vi "input.vi"(8 "error in":errorcluster, 10 "data table in":T1, 11 "OPC UA runtime in":refnum<class "OPC UA runtime.lvclass">) -> (0 "error out":errorcluster, 2 "data table out":T1, 3 "OPC UA runtime out":refnum<class "OPC UA runtime.lvclass">)   [LabVIEW 2013, in "OPC UA runtime.lvclass"]
doc: "Provides an interface for reading data from a module at runtime. While this interface performs no operations, a child should provide an override which may read from any open sessions, references, or interfaces."
uses:
  OPC UA runtime.lvclass
  <vilib>/NI/Tag Bus/table/data table.lvlib
  <vilib>/opcua/NI OPC UA Client.lvlib
  <vilib>/OPCUA/client/Read Bool.vi
  <vilib>/NI/Tag Bus/table/data polymorphs/write one/write Boolean.vi
  <vilib>/NI/Tag Bus/table/data polymorphs/write one/write String.vi
  <vilib>/NI/Tag Bus/table/data polymorphs/write one/write Array of String.vi
  <vilib>/OPCUA/client/Read UInt16.vi
  <vilib>/OPCUA/client/Read Int32.vi
  <vilib>/OPCUA/client/Read ByteString Array.vi
  <vilib>/OPCUA/client/Read SByte.vi
  <vilib>/OPCUA/client/Read String Array.vi
  <vilib>/OPCUA/client/Read UInt32.vi
  <vilib>/OPCUA/client/Read Double.vi
  <vilib>/OPCUA/client/Read Float.vi
  <vilib>/OPCUA/client/Read Int64.vi
  <vilib>/OPCUA/client/Read UInt64.vi
  <vilib>/OPCUA/client/Read Double Array.vi
  <vilib>/OPCUA/client/Read Int16 Array.vi
  <vilib>/OPCUA/client/Read Byte Array.vi
  <vilib>/OPCUA/client/Read UInt64 Array.vi
  <vilib>/OPCUA/client/Read Int32 Array.vi
  <vilib>/OPCUA/client/Read ByteString.vi
  <vilib>/OPCUA/client/Read UInt32 Array.vi
  <vilib>/OPCUA/client/Read SByte Array.vi
  <vilib>/OPCUA/client/Read UInt16 Array.vi
  <vilib>/OPCUA/client/Read Int16.vi
  <vilib>/OPCUA/client/Read String.vi
  <vilib>/OPCUA/client/Read Int64 Array.vi
  <vilib>/OPCUA/client/Read Byte.vi
  <vilib>/OPCUA/client/Read Float Array.vi
  <vilib>/OPCUA/client/Read Bool Array.vi
  <vilib>/NI/Tag Bus/table/data polymorphs/write one/write I16.vi
  <vilib>/NI/Tag Bus/table/data polymorphs/write one/write U16.vi
  <vilib>/NI/Tag Bus/table/data polymorphs/write one/write I32.vi
  <vilib>/NI/Tag Bus/table/data polymorphs/write one/write Array of I64.vi
  <vilib>/NI/Tag Bus/table/data polymorphs/write one/write Array of I16.vi
  <vilib>/NI/Tag Bus/table/data polymorphs/write one/write Single.vi
  <vilib>/NI/Tag Bus/table/data polymorphs/write one/write I64.vi
  <vilib>/NI/Tag Bus/table/data polymorphs/write one/write U32.vi
  <vilib>/NI/Tag Bus/table/data polymorphs/write one/write U64.vi
  <vilib>/NI/Tag Bus/table/data polymorphs/write one/write U8.vi
  <vilib>/NI/Tag Bus/table/data polymorphs/write one/write Array of I8.vi
  <vilib>/NI/Tag Bus/table/data polymorphs/write one/write Array of U16.vi
  <vilib>/NI/Tag Bus/table/data polymorphs/write one/write I8.vi
  <vilib>/NI/Tag Bus/table/data polymorphs/write one/write Array of U32.vi
  <vilib>/NI/Tag Bus/table/data polymorphs/write one/write Array of I32.vi
  <vilib>/NI/Tag Bus/table/data polymorphs/write one/write Array of Boolean.vi
  <vilib>/NI/Tag Bus/table/data polymorphs/write one/write Array of U8.vi
  <vilib>/NI/Tag Bus/table/data polymorphs/write one/write Array of Single.vi
  <vilib>/NI/Tag Bus/table/data polymorphs/write one/write Array of Double.vi
  <vilib>/NI/Tag Bus/table/data polymorphs/write one/write Array of U64.vi
  <vilib>/NI/Tag Bus/table/data polymorphs/write one/write Double.vi
  <vilib>/OPCUA/client/Read DateTime.vi
  <vilib>/OPCUA/client/Read DateTime Array.vi
  <vilib>/opcua/NI OPC UA Server.lvlib
  <vilib>/OPCUA/server/Read Bool.vi
  <vilib>/OPCUA/server/Read SByte.vi
  <vilib>/OPCUA/server/Read Byte.vi
  <vilib>/OPCUA/server/Read Int16.vi
  <vilib>/OPCUA/server/Read UInt16.vi
  <vilib>/OPCUA/server/Read Int32.vi
  <vilib>/OPCUA/server/Read UInt32.vi
  <vilib>/OPCUA/server/Read Int64.vi
  <vilib>/OPCUA/server/Read UInt64.vi
  <vilib>/OPCUA/server/Read Float.vi
  <vilib>/OPCUA/server/Read Double.vi
  <vilib>/OPCUA/server/Read String.vi
  <vilib>/OPCUA/server/Read Date Time.vi
  <vilib>/OPCUA/server/Read Byte String.vi
  <vilib>/OPCUA/server/Read Bool Array.vi
  <vilib>/OPCUA/server/Read SByte Array.vi
  <vilib>/OPCUA/server/Read Byte Array.vi
  <vilib>/OPCUA/server/Read Int16 Array.vi
  <vilib>/OPCUA/server/Read UInt16 Array.vi
  <vilib>/OPCUA/server/Read Int32 Array.vi
  <vilib>/OPCUA/server/Read UInt32 Array.vi
  <vilib>/OPCUA/server/Read Int64 Array.vi
  <vilib>/OPCUA/server/Read UInt64 Array.vi
  <vilib>/OPCUA/server/Read Float Array.vi
  <vilib>/OPCUA/server/Read Double Array.vi
  <vilib>/OPCUA/server/Read String Array.vi
  <vilib>/OPCUA/server/Read Date Time Array.vi
  <vilib>/OPCUA/server/Read Byte String Array.vi
  <vilib>/NI/Tag Bus/table/data table.ctl
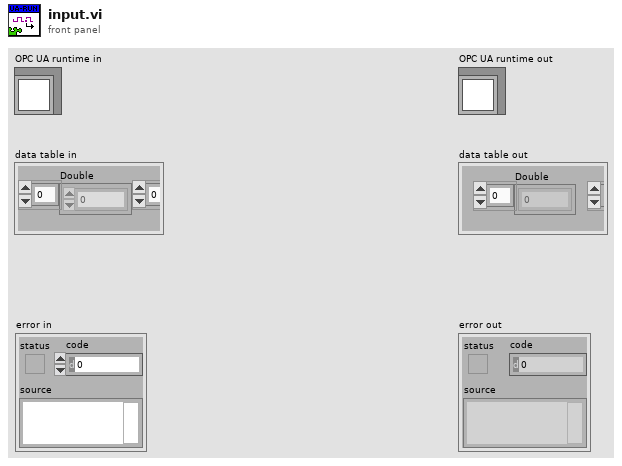
[diagram p1: front panel]
types:
  T1 = typedef "tag bus.lvlib/data table.lvlib/data table.ctl" = cluster{"Double":dbl[], "Single":sgl[], "I64":i64[], "I32":i32[], "I16":i16[], "I8":i8[], "U64":u64[], "U32":u32[], "U16":u16[], "U8":u8[], "Boolean":bool[], "String":string[], "Array of Double":cluster{"DBL Array":dbl[]}[], "Array of Single":cluster{"SGL Array":sgl[]}[], "Array of I64":cluster{"I64 Array":i64[]}[], "Array of I32":cluster{"I32 Array":i32[]}[], "Array of I16":cluster{"I16 Array":i16[]}[], "Array of I8":cluster{"I8 Array":i8[]}[], "Array of U64":cluster{"U64 Array":u64[]}[], "Array of U32":cluster{"U32 Array":u32[]}[], "Array of U16":cluster{"U16 Array":u16[]}[], "Array of U8":cluster{"U8 Array":u8[]}[], "Array of Boolean":cluster{"Boolean Array":bool[]}[], "Array of String":cluster{"String Array":string[]}[]}
  T2 = typedef "tag bus.lvlib/tag descriptor.lvclass/Data Type.ctl" = enum16{"Double", "Single", "I64", "I32", "I16", "I8", "U64", "U32", "U16", "U8", "Boolean", "String", "Array of Double", "Array of Single", "Array of I64", "Array of I32", "Array of I16", "Array of I8", "Array of U64", "Array of U32", "Array of U16", "Array of U8", "Array of Boolean", "Array of String"}
  T3 = typedef "OPC UA configuration.lvclass/OPC UA Data Type.ctl" = u16
  T4 = cluster{"DCAF Data Type":T2, "Index":i32, "Node Path":string, "OPC UA Data Type":T3}[]
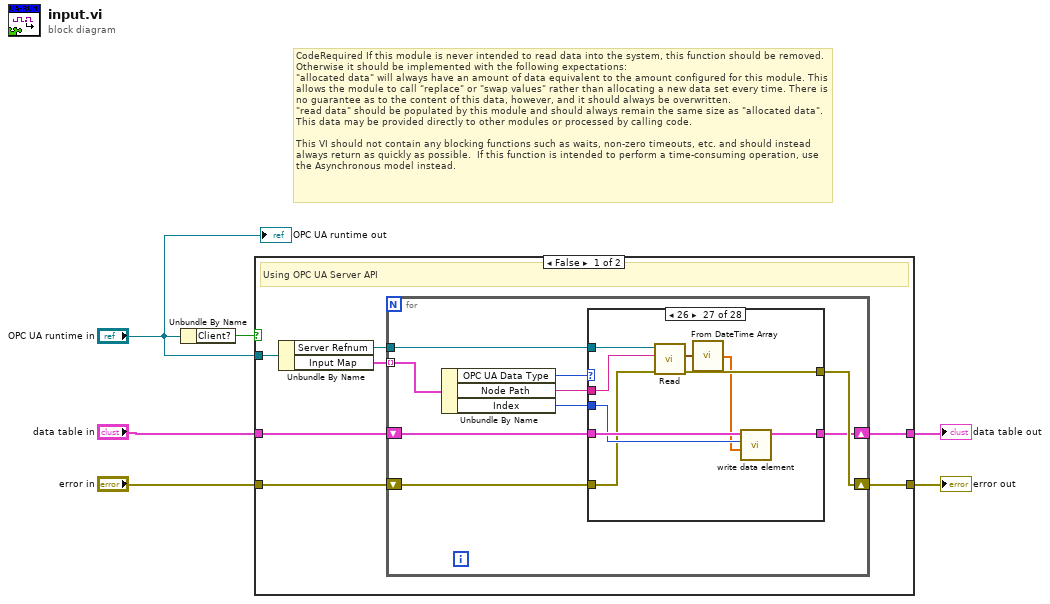
[diagram p0: block diagram]
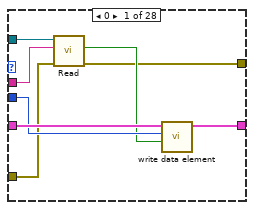
[diagram p2: hidden frame]
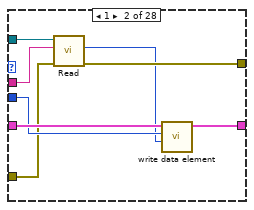
[diagram p3: hidden frame]
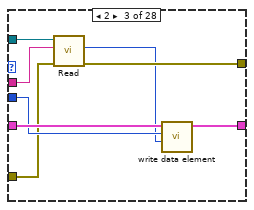
[diagram p4: hidden frame]
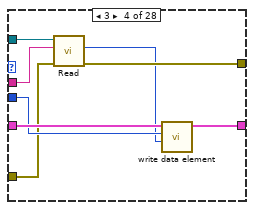
[diagram p5: hidden frame]
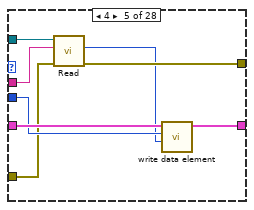
[diagram p6: hidden frame]
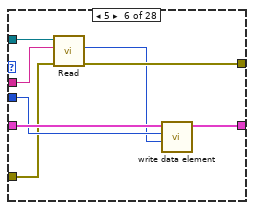
[diagram p7: hidden frame]
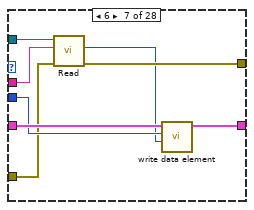
[diagram p8: hidden frame]
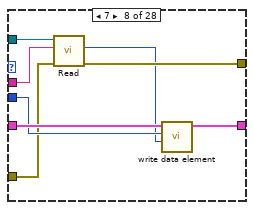
[diagram p9: hidden frame]
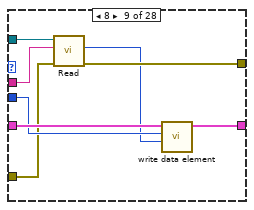
[diagram p10: hidden frame]
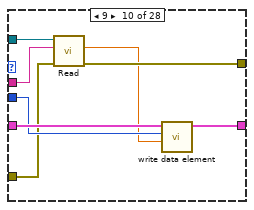
[diagram p11: hidden frame]
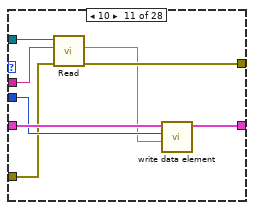
[diagram p12: hidden frame]
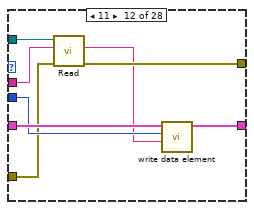
[diagram p13: hidden frame]
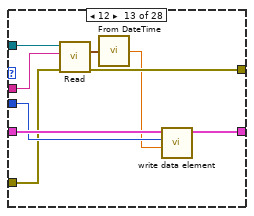
[diagram p14: hidden frame]
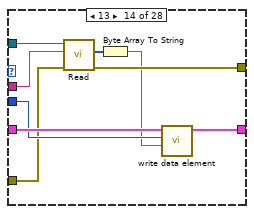
[diagram p15: hidden frame]
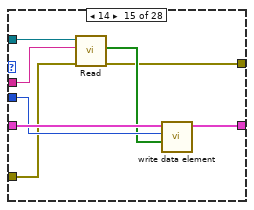
[diagram p16: hidden frame]
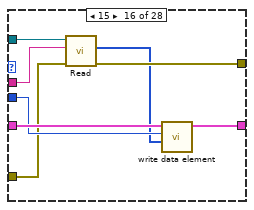
[diagram p17: hidden frame]
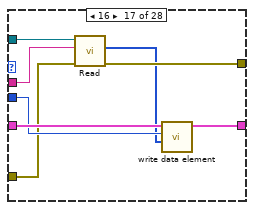
[diagram p18: hidden frame]
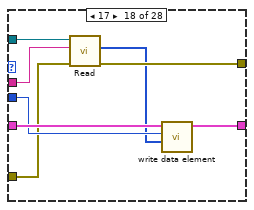
[diagram p19: hidden frame]
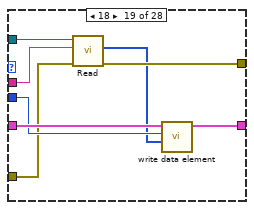
[diagram p20: hidden frame]
diagram:
  # "CodeRequired If this module is never intended to read data into the system, this function should be removed. Otherwise it should be implemented with the following expectations:\n\"allocated data\" will always have an amount of data equivalent to the amount configured for this module. This allows the module to call \"replace\" or \"swap values\" rather than allocating a new data set every time. There is no guarantee as to the content of this data, however, and it should always be overwritten.\n\"read data\" should be populated by this module and should always remain the same size as \"allocated data\". This data may be provided directly to other modules or processed by calling code.\n\nThis VI should not contain any blocking functions such as waits, non-zero timeouts, etc. and should instead always return as quickly as possible.  If this function is intended to perform a time-consuming operation, use the Asynchronous model instead."
  n1 = Unbundle By Name("OPC UA runtime in") -> ("Client?"=w6:bool)
  n2 = case shown="False" w6 {
    tunnel: "OPC UA runtime in" -> [w13 w259]
    tunnel: "data table in" -> [w9 w256]
    tunnel: "error in" -> [w8 w255]
    tunnel: [w10 w254] -> w2
    tunnel: [w7 w253] -> w1
    frame False {
      # "Using OPC UA Server API"
      n3 = Unbundle By Name(w13) -> ("Server Refnum"=w11:refnum<k21>, "Input Map"=w12:T4)
      n4 = for {
        tunnel: w11 -> [w18]
        tunnel: w12 -> [w22] mode=indexing
        shift-right: [w15] -> w7
        shift-left: w8 -> [w16]
        shift-right: [w14] -> w10
        shift-left: w9 -> [w17]
        n5 = Unbundle By Name(w22) -> ("OPC UA Data Type"=w21:T3, "Node Path"=w20:string, "Index"=w19:i32)
        n6 = case shown="26" w21 {
          tunnel: w20 -> [w29 w37 w45 w53 w61 w69 w77 w85 w93 w101 w109 w117 w126 w135 w144 w152 w160 w168 w176 w184 w192 w200 w208 w216 w224 w232 w241 w249]
          tunnel: w19 -> [w27 w35 w43 w51 w59 w67 w75 w83 w91 w99 w107 w115 w124 w133 w142 w150 w158 w166 w174 w182 w190 w198 w206 w214 w222 w230 w239 w247]
          tunnel: w18 -> [w30 w38 w46 w54 w62 w70 w78 w86 w94 w102 w110 w118 w127 w136 w137 w146 w153 w162 w170 w178 w186 w194 w202 w210 w218 w225 w234 w250]
          tunnel: w17 -> [w28 w36 w44 w52 w60 w68 w76 w84 w92 w100 w108 w116 w125 w134 w143 w151 w159 w167 w175 w183 w191 w199 w207 w215 w223 w231 w240 w248]
          tunnel: w16 -> [w25 w34 w42 w50 w58 w66 w74 w82 w90 w98 w106 w114 w123 w132 w140 w149 w157 w165 w173 w181 w189 w197 w205 w213 w221 w228 w238 w246]
          tunnel: [w24 w33 w41 w49 w57 w65 w73 w81 w89 w97 w105 w113 w122 w131 w139 w148 w156 w164 w172 w180 w188 w196 w204 w212 w220 w227 w237 w245] -> w15
          tunnel: [w23 w32 w40 w48 w56 w64 w72 w80 w88 w96 w104 w112 w121 w130 w138 w147 w155 w163 w171 w179 w187 w195 w203 w211 w219 w226 w236 w244] -> w14
          frame 0 {
            n7 = call-poly <vilib>:"Read.vi"("error in (no error)"=w25, "node path"=w29, "OPC UA server refnum in"=w30) -> ("error out"=w24:errorcluster, "value"=w26:bool)  [unwired: 4 in, 3 out]
            n8 = call-poly <vilib>:"write data element.vi"("value"=w26, "index"=w27, "data table in"=w28) -> ("data table out"=w23:T1)  [unwired: 8 in]
          }
          frame 1 {
            n9 = call-poly <vilib>:"Read.vi"("error in (no error)"=w34, "node path"=w37, "OPC UA server refnum in"=w38) -> ("error out"=w33:errorcluster, "value"=w31:i8)  [unwired: 4 in, 3 out]
            n10 = call-poly <vilib>:"write data element.vi"("value"=w31, "index"=w35, "data table in"=w36) -> ("data table out"=w32:T1)  [unwired: 8 in]
          }
          frame 2 {
            n11 = call-poly <vilib>:"Read.vi"("error in (no error)"=w42, "node path"=w45, "OPC UA server refnum in"=w46) -> ("error out"=w41:errorcluster, "value"=w39:u8)  [unwired: 4 in, 3 out]
            n12 = call-poly <vilib>:"write data element.vi"("value"=w39, "index"=w43, "data table in"=w44) -> ("data table out"=w40:T1)  [unwired: 8 in]
          }
          frame 3 {
            n13 = call-poly <vilib>:"Read.vi"("error in (no error)"=w50, "node path"=w53, "OPC UA server refnum in"=w54) -> ("error out"=w49:errorcluster, "value"=w47:i16)  [unwired: 4 in, 3 out]
            n14 = call-poly <vilib>:"write data element.vi"("value"=w47, "index"=w51, "data table in"=w52) -> ("data table out"=w48:T1)  [unwired: 8 in]
          }
          frame 4 {
            n15 = call-poly <vilib>:"Read.vi"("error in (no error)"=w58, "node path"=w61, "OPC UA server refnum in"=w62) -> ("error out"=w57:errorcluster, "value"=w55:u16)  [unwired: 4 in, 3 out]
            n16 = call-poly <vilib>:"write data element.vi"("value"=w55, "index"=w59, "data table in"=w60) -> ("data table out"=w56:T1)  [unwired: 8 in]
          }
          frame 5 {
            n17 = call-poly <vilib>:"Read.vi"("error in (no error)"=w66, "node path"=w69, "OPC UA server refnum in"=w70) -> ("error out"=w65:errorcluster, "value"=w63:i32)  [unwired: 4 in, 3 out]
            n18 = call-poly <vilib>:"write data element.vi"("value"=w63, "index"=w67, "data table in"=w68) -> ("data table out"=w64:T1)  [unwired: 8 in]
          }
          frame 6 {
            n19 = call-poly <vilib>:"Read.vi"("error in (no error)"=w74, "node path"=w77, "OPC UA server refnum in"=w78) -> ("error out"=w73:errorcluster, "value"=w71:u32)  [unwired: 4 in, 3 out]
            n20 = call-poly <vilib>:"write data element.vi"("value"=w71, "index"=w75, "data table in"=w76) -> ("data table out"=w72:T1)  [unwired: 8 in]
          }
          frame 7 {
            n21 = call-poly <vilib>:"Read.vi"("error in (no error)"=w82, "node path"=w85, "OPC UA server refnum in"=w86) -> ("error out"=w81:errorcluster, "value"=w79:i64)  [unwired: 4 in, 3 out]
            n22 = call-poly <vilib>:"write data element.vi"("value"=w79, "index"=w83, "data table in"=w84) -> ("data table out"=w80:T1)  [unwired: 8 in]
          }
          frame 8 {
            n23 = call-poly <vilib>:"Read.vi"("error in (no error)"=w90, "node path"=w93, "OPC UA server refnum in"=w94) -> ("error out"=w89:errorcluster, "value"=w87:u64)  [unwired: 4 in, 3 out]
            n24 = call-poly <vilib>:"write data element.vi"("value"=w87, "index"=w91, "data table in"=w92) -> ("data table out"=w88:T1)  [unwired: 8 in]
          }
          frame 9 {
            n25 = call-poly <vilib>:"Read.vi"("error in (no error)"=w98, "node path"=w101, "OPC UA server refnum in"=w102) -> ("error out"=w97:errorcluster, "value"=w95:sgl)  [unwired: 4 in, 3 out]
            n26 = call-poly <vilib>:"write data element.vi"("value"=w95, "index"=w99, "data table in"=w100) -> ("data table out"=w96:T1)  [unwired: 8 in]
          }
          frame 10 {
            n27 = call-poly <vilib>:"Read.vi"("error in (no error)"=w106, "node path"=w109, "OPC UA server refnum in"=w110) -> ("error out"=w105:errorcluster, "value"=w103:dbl)  [unwired: 4 in, 3 out]
            n28 = call-poly <vilib>:"write data element.vi"("value"=w103, "index"=w107, "data table in"=w108) -> ("data table out"=w104:T1)  [unwired: 8 in]
          }
          frame 11 {
            n29 = call-poly <vilib>:"Read.vi"("error in (no error)"=w114, "node path"=w117, "OPC UA server refnum in"=w118) -> ("error out"=w113:errorcluster, "value"=w111:string)  [unwired: 4 in, 3 out]
            n30 = call-poly <vilib>:"write data element.vi"("value"=w111, "index"=w115, "data table in"=w116) -> ("data table out"=w112:T1)  [unwired: 8 in]
          }
          frame 12 {
            n31 = call-poly <vilib>:"Read.vi"("error in (error in)"=w123, "node path"=w126, "OPC UA server refnum in"=w127) -> ("error out"=w122:errorcluster, "timestamp"=w120:timestamp)  [unwired: 4 in, 3 out]
            n32 = call "From DateTime.vi"("DateTime"=w120) -> ("Formatted DateTime"=w119:dbl)
            n33 = call-poly <vilib>:"write data element.vi"("value"=w119, "index"=w124, "data table in"=w125) -> ("data table out"=w121:T1)  [unwired: 8 in]
          }
          frame 13 {
            n34 = call-poly <vilib>:"Read.vi"("error in (no error)"=w132, "node path"=w135, "OPC UA server refnum in"=w136) -> ("error out"=w131:errorcluster, "value"=w128:u8[])  [unwired: 4 in, 3 out]
            n35 = Byte Array To String(unsigned byte array=w128) -> (string=w129:string)
            n36 = call-poly <vilib>:"write data element.vi"("value"=w129, "index"=w133, "data table in"=w134) -> ("data table out"=w130:T1)  [unwired: 8 in]
          }
          frame 14 {
            n37 = call-poly <vilib>:"Read.vi"("error in (no error)"=w140, "node path"=w144, "OPC UA server refnum in"=w137) -> ("error out"=w139:errorcluster, "value"=w141:bool[])  [unwired: 4 in, 3 out]
            n38 = call-poly <vilib>:"write data element.vi"("value"=w141, "index"=w142, "data table in"=w143) -> ("data table out"=w138:T1)  [unwired: 8 in]
          }
          frame 15 {
            n39 = call-poly <vilib>:"Read.vi"("error in (no error)"=w149, "node path"=w152, "OPC UA server refnum in"=w146) -> ("error out"=w148:errorcluster, "value"=w145:i8[])  [unwired: 4 in, 3 out]
            n40 = call-poly <vilib>:"write data element.vi"("value"=w145, "index"=w150, "data table in"=w151) -> ("data table out"=w147:T1)  [unwired: 8 in]
          }
          frame 16 {
            n41 = call-poly <vilib>:"Read.vi"("error in (no error)"=w157, "node path"=w160, "OPC UA server refnum in"=w153) -> ("error out"=w156:errorcluster, "value"=w154:u8[])  [unwired: 4 in, 3 out]
            n42 = call-poly <vilib>:"write data element.vi"("value"=w154, "index"=w158, "data table in"=w159) -> ("data table out"=w155:T1)  [unwired: 8 in]
          }
          frame 17 {
            n43 = call-poly <vilib>:"Read.vi"("error in (no error)"=w165, "node path"=w168, "OPC UA server refnum in"=w162) -> ("error out"=w164:errorcluster, "value"=w161:i16[])  [unwired: 4 in, 3 out]
            n44 = call-poly <vilib>:"write data element.vi"("value"=w161, "index"=w166, "data table in"=w167) -> ("data table out"=w163:T1)  [unwired: 8 in]
          }
          frame 18 {
            n45 = call-poly <vilib>:"Read.vi"("error in (no error)"=w173, "node path"=w176, "OPC UA server refnum in"=w170) -> ("error out"=w172:errorcluster, "value"=w169:u16[])  [unwired: 4 in, 3 out]
            n46 = call-poly <vilib>:"write data element.vi"("value"=w169, "index"=w174, "data table in"=w175) -> ("data table out"=w171:T1)  [unwired: 8 in]
          }
          frame 19 {
            n47 = call-poly <vilib>:"Read.vi"("error in (no error)"=w181, "node path"=w184, "OPC UA server refnum in"=w178) -> ("error out"=w180:errorcluster, "value"=w177:i32[])  [unwired: 4 in, 3 out]
            n48 = call-poly <vilib>:"write data element.vi"("value"=w177, "index"=w182, "data table in"=w183) -> ("data table out"=w179:T1)  [unwired: 8 in]
          }
          frame 20 {
            n49 = call-poly <vilib>:"Read.vi"("error in (no error)"=w189, "node path"=w192, "OPC UA server refnum in"=w186) -> ("error out"=w188:errorcluster, "value"=w185:u32[])  [unwired: 4 in, 3 out]
            n50 = call-poly <vilib>:"write data element.vi"("value"=w185, "index"=w190, "data table in"=w191) -> ("data table out"=w187:T1)  [unwired: 8 in]
          }
          frame 21 {
            n51 = call-poly <vilib>:"Read.vi"("error in (no error)"=w197, "node path"=w200, "OPC UA server refnum in"=w194) -> ("error out"=w196:errorcluster, "value"=w193:i64[])  [unwired: 4 in, 3 out]
            n52 = call-poly <vilib>:"write data element.vi"("value"=w193, "index"=w198, "data table in"=w199) -> ("data table out"=w195:T1)  [unwired: 8 in]
          }
          frame 22 {
            n53 = call-poly <vilib>:"Read.vi"("error in (no error)"=w205, "node path"=w208, "OPC UA server refnum in"=w202) -> ("error out"=w204:errorcluster, "value"=w201:u64[])  [unwired: 4 in, 3 out]
            n54 = call-poly <vilib>:"write data element.vi"("value"=w201, "index"=w206, "data table in"=w207) -> ("data table out"=w203:T1)  [unwired: 8 in]
          }
          frame 23 {
            n55 = call-poly <vilib>:"Read.vi"("error in (no error)"=w213, "node path"=w216, "OPC UA server refnum in"=w210) -> ("error out"=w212:errorcluster, "value"=w209:sgl[])  [unwired: 4 in, 3 out]
            n56 = call-poly <vilib>:"write data element.vi"("value"=w209, "index"=w214, "data table in"=w215) -> ("data table out"=w211:T1)  [unwired: 8 in]
          }
          frame 24 {
            n57 = call-poly <vilib>:"Read.vi"("error in (no error)"=w221, "node path"=w224, "OPC UA server refnum in"=w218) -> ("error out"=w220:errorcluster, "value"=w217:dbl[])  [unwired: 4 in, 3 out]
            n58 = call-poly <vilib>:"write data element.vi"("value"=w217, "index"=w222, "data table in"=w223) -> ("data table out"=w219:T1)  [unwired: 8 in]
          }
          frame 25 {
            n59 = call-poly <vilib>:"Read.vi"("error in (no error)"=w228, "node path"=w232, "OPC UA server refnum in"=w225) -> ("error out"=w227:errorcluster, "value"=w229:string[])  [unwired: 4 in, 3 out]
            n60 = call-poly <vilib>:"write data element.vi"("value"=w229, "index"=w230, "data table in"=w231) -> ("data table out"=w226:T1)  [unwired: 8 in]
          }
          frame 26 {
            n61 = call-poly <vilib>:"Read.vi"("error in (no error)"=w238, "node path"=w241, "OPC UA server refnum in"=w234) -> ("error out"=w237:errorcluster, "value"=w233:timestamp[])  [unwired: 4 in, 3 out]
            n62 = call "From DateTime Array.vi"("DateTime Array"=w233) -> ("Formatted DateTime Array"=w235:dbl[])
            n63 = call-poly <vilib>:"write data element.vi"("value"=w235, "index"=w239, "data table in"=w240) -> ("data table out"=w236:T1)  [unwired: 8 in]
          }
          frame 27 {
            n64 = call-poly <vilib>:"Read.vi"("error in (no error)"=w246, "node path"=w249, "OPC UA server refnum in"=w250) -> ("error out"=w245:errorcluster, "value"=w242:u8[][])  [unwired: 4 in, 3 out]
            n65 = for {
              tunnel: [w252] -> w243 mode=indexing
              tunnel: w242 -> [w251] mode=indexing
              n66 = Byte Array To String(unsigned byte array=w251) -> (string=w252:string)
            }
            n67 = call-poly <vilib>:"write data element.vi"("value"=w243, "index"=w247, "data table in"=w248) -> ("data table out"=w244:T1)  [unwired: 8 in]
          }
        }
      }
    }
    frame True {
      # "Using OPC UA Client API"
      n68 = Unbundle By Name(w259) -> ("Client Refnum"=w258:refnum<k21>, "Input Map"=w257:T4)
      n69 = for {
        tunnel: w258 -> [w264]
        tunnel: w257 -> [w268] mode=indexing
        shift-right: [w261] -> w253
        shift-left: w255 -> [w262]
        shift-right: [w260] -> w254
        shift-left: w256 -> [w263]
        n70 = Unbundle By Name(w268) -> ("OPC UA Data Type"=w267:T3, "Node Path"=w266:string, "Index"=w265:i32)
        n71 = case shown="1" w267 {
          tunnel: w266 -> [w275 w283 w291 w299 w307 w315 w323 w331 w339 w347 w355 w363 w372 w381 w389 w397 w405 w413 w421 w429 w437 w445 w453 w461 w469 w477 w486 w495]
          tunnel: w265 -> [w273 w281 w289 w297 w305 w313 w321 w329 w337 w345 w353 w361 w370 w379 w387 w395 w403 w411 w419 w427 w435 w443 w451 w459 w467 w475 w484 w493]
          tunnel: w264 -> [w276 w284 w292 w300 w308 w316 w324 w332 w340 w348 w356 w364 w373 w382 w390 w398 w406 w414 w422 w430 w438 w446 w454 w462 w470 w478 w487 w496]
          tunnel: w263 -> [w274 w282 w290 w298 w306 w314 w322 w330 w338 w346 w354 w362 w371 w380 w388 w396 w404 w412 w420 w428 w436 w444 w452 w460 w468 w476 w485 w494]
          tunnel: w262 -> [w271 w279 w287 w295 w303 w311 w319 w327 w335 w343 w351 w359 w369 w378 w385 w393 w401 w409 w417 w425 w433 w441 w449 w457 w465 w473 w483 w492]
          tunnel: [w270 w278 w286 w294 w302 w310 w318 w326 w334 w342 w350 w358 w368 w377 w384 w392 w400 w408 w416 w424 w432 w440 w448 w456 w464 w472 w482 w491] -> w261
          tunnel: [w269 w277 w285 w293 w301 w309 w317 w325 w333 w341 w349 w357 w367 w376 w383 w391 w399 w407 w415 w423 w431 w439 w447 w455 w463 w471 w481 w490] -> w260
          frame 0 {
            n72 = call-poly <vilib>:"Read.vi"("error in (no error)"=w271, "node path"=w275, "OPC UA client refnum in"=w276) -> ("error out"=w270:errorcluster, "value"=w272:bool)  [unwired: 4 in, 3 out]
            n73 = call-poly <vilib>:"write data element.vi"("value"=w272, "index"=w273, "data table in"=w274) -> ("data table out"=w269:T1)  [unwired: 8 in]
          }
          frame 1 {
            n74 = call-poly <vilib>:"Read.vi"("error in (no error)"=w279, "node path"=w283, "OPC UA client refnum in"=w284) -> ("error out"=w278:errorcluster, "value"=w280:i8)  [unwired: 4 in, 3 out]
            n75 = call-poly <vilib>:"write data element.vi"("value"=w280, "index"=w281, "data table in"=w282) -> ("data table out"=w277:T1)  [unwired: 8 in]
          }
          frame 2 {
            n76 = call-poly <vilib>:"Read.vi"("error in (no error)"=w287, "node path"=w291, "OPC UA client refnum in"=w292) -> ("error out"=w286:errorcluster, "value"=w288:u8)  [unwired: 4 in, 3 out]
            n77 = call-poly <vilib>:"write data element.vi"("value"=w288, "index"=w289, "data table in"=w290) -> ("data table out"=w285:T1)  [unwired: 8 in]
          }
          frame 3 {
            n78 = call-poly <vilib>:"Read.vi"("error in (no error)"=w295, "node path"=w299, "OPC UA client refnum in"=w300) -> ("error out"=w294:errorcluster, "value"=w296:i16)  [unwired: 4 in, 3 out]
            n79 = call-poly <vilib>:"write data element.vi"("value"=w296, "index"=w297, "data table in"=w298) -> ("data table out"=w293:T1)  [unwired: 8 in]
          }
          frame 4 {
            n80 = call-poly <vilib>:"Read.vi"("error in (no error)"=w303, "node path"=w307, "OPC UA client refnum in"=w308) -> ("error out"=w302:errorcluster, "value"=w304:u16)  [unwired: 4 in, 3 out]
            n81 = call-poly <vilib>:"write data element.vi"("value"=w304, "index"=w305, "data table in"=w306) -> ("data table out"=w301:T1)  [unwired: 8 in]
          }
          frame 5 {
            n82 = call-poly <vilib>:"Read.vi"("error in (no error)"=w311, "node path"=w315, "OPC UA client refnum in"=w316) -> ("error out"=w310:errorcluster, "value"=w312:i32)  [unwired: 4 in, 3 out]
            n83 = call-poly <vilib>:"write data element.vi"("value"=w312, "index"=w313, "data table in"=w314) -> ("data table out"=w309:T1)  [unwired: 8 in]
          }
          frame 6 {
            n84 = call-poly <vilib>:"Read.vi"("error in (no error)"=w319, "node path"=w323, "OPC UA client refnum in"=w324) -> ("error out"=w318:errorcluster, "value"=w320:u32)  [unwired: 4 in, 3 out]
            n85 = call-poly <vilib>:"write data element.vi"("value"=w320, "index"=w321, "data table in"=w322) -> ("data table out"=w317:T1)  [unwired: 8 in]
          }
          frame 7 {
            n86 = call-poly <vilib>:"Read.vi"("error in (no error)"=w327, "node path"=w331, "OPC UA client refnum in"=w332) -> ("error out"=w326:errorcluster, "value"=w328:i64)  [unwired: 4 in, 3 out]
            n87 = call-poly <vilib>:"write data element.vi"("value"=w328, "index"=w329, "data table in"=w330) -> ("data table out"=w325:T1)  [unwired: 8 in]
          }
          frame 8 {
            n88 = call-poly <vilib>:"Read.vi"("error in (no error)"=w335, "node path"=w339, "OPC UA client refnum in"=w340) -> ("error out"=w334:errorcluster, "value"=w336:u64)  [unwired: 4 in, 3 out]
            n89 = call-poly <vilib>:"write data element.vi"("value"=w336, "index"=w337, "data table in"=w338) -> ("data table out"=w333:T1)  [unwired: 8 in]
          }
          frame 9 {
            n90 = call-poly <vilib>:"Read.vi"("error in (no error)"=w343, "node path"=w347, "OPC UA client refnum in"=w348) -> ("error out"=w342:errorcluster, "value"=w344:sgl)  [unwired: 4 in, 3 out]
            n91 = call-poly <vilib>:"write data element.vi"("value"=w344, "index"=w345, "data table in"=w346) -> ("data table out"=w341:T1)  [unwired: 8 in]
          }
          frame 10 {
            n92 = call-poly <vilib>:"Read.vi"("error in (no error)"=w351, "node path"=w355, "OPC UA client refnum in"=w356) -> ("error out"=w350:errorcluster, "value"=w352:dbl)  [unwired: 4 in, 3 out]
            n93 = call-poly <vilib>:"write data element.vi"("value"=w352, "index"=w353, "data table in"=w354) -> ("data table out"=w349:T1)  [unwired: 8 in]
          }
          frame 11 {
            n94 = call-poly <vilib>:"Read.vi"("error in (no error)"=w359, "node path"=w363, "OPC UA client refnum in"=w364) -> ("error out"=w358:errorcluster, "value"=w360:string)  [unwired: 4 in, 3 out]
            n95 = call-poly <vilib>:"write data element.vi"("value"=w360, "index"=w361, "data table in"=w362) -> ("data table out"=w357:T1)  [unwired: 8 in]
          }
          frame 12 {
            n96 = call-poly <vilib>:"Read.vi"("error in (no error)"=w369, "node path"=w372, "OPC UA client refnum in"=w373) -> ("error out"=w368:errorcluster, "value"=w366:timestamp)  [unwired: 4 in, 3 out]
            n97 = call "From DateTime.vi"("DateTime"=w366) -> ("Formatted DateTime"=w365:dbl)
            n98 = call-poly <vilib>:"write data element.vi"("value"=w365, "index"=w370, "data table in"=w371) -> ("data table out"=w367:T1)  [unwired: 8 in]
          }
          frame 13 {
            n99 = call-poly <vilib>:"Read.vi"("error in (no error)"=w378, "node path"=w381, "OPC UA client refnum in"=w382) -> ("error out"=w377:errorcluster, "value"=w375:u8[])  [unwired: 4 in, 3 out]
            n100 = Byte Array To String(unsigned byte array=w375) -> (string=w374:string)
            n101 = call-poly <vilib>:"write data element.vi"("value"=w374, "index"=w379, "data table in"=w380) -> ("data table out"=w376:T1)  [unwired: 8 in]
          }
          frame 14 {
            n102 = call-poly <vilib>:"Read.vi"("error in (no error)"=w385, "node path"=w389, "OPC UA client refnum in"=w390) -> ("error out"=w384:errorcluster, "value"=w386:bool[])  [unwired: 4 in, 3 out]
            n103 = call-poly <vilib>:"write data element.vi"("value"=w386, "index"=w387, "data table in"=w388) -> ("data table out"=w383:T1)  [unwired: 8 in]
          }
          frame 15 {
            n104 = call-poly <vilib>:"Read.vi"("error in (no error)"=w393, "node path"=w397, "OPC UA client refnum in"=w398) -> ("error out"=w392:errorcluster, "value"=w394:i8[])  [unwired: 4 in, 3 out]
            n105 = call-poly <vilib>:"write data element.vi"("value"=w394, "index"=w395, "data table in"=w396) -> ("data table out"=w391:T1)  [unwired: 8 in]
          }
          frame 16 {
            n106 = call-poly <vilib>:"Read.vi"("error in (no error)"=w401, "node path"=w405, "OPC UA client refnum in"=w406) -> ("error out"=w400:errorcluster, "value"=w402:u8[])  [unwired: 4 in, 3 out]
            n107 = call-poly <vilib>:"write data element.vi"("value"=w402, "index"=w403, "data table in"=w404) -> ("data table out"=w399:T1)  [unwired: 8 in]
          }
          frame 17 {
            n108 = call-poly <vilib>:"Read.vi"("error in (no error)"=w409, "node path"=w413, "OPC UA client refnum in"=w414) -> ("error out"=w408:errorcluster, "value"=w410:i16[])  [unwired: 4 in, 3 out]
            n109 = call-poly <vilib>:"write data element.vi"("value"=w410, "index"=w411, "data table in"=w412) -> ("data table out"=w407:T1)  [unwired: 8 in]
          }
          frame 18 {
            n110 = call-poly <vilib>:"Read.vi"("error in (no error)"=w417, "node path"=w421, "OPC UA client refnum in"=w422) -> ("error out"=w416:errorcluster, "value"=w418:u16[])  [unwired: 4 in, 3 out]
            n111 = call-poly <vilib>:"write data element.vi"("value"=w418, "index"=w419, "data table in"=w420) -> ("data table out"=w415:T1)  [unwired: 8 in]
          }
          frame 19 {
            n112 = call-poly <vilib>:"Read.vi"("error in (no error)"=w425, "node path"=w429, "OPC UA client refnum in"=w430) -> ("error out"=w424:errorcluster, "value"=w426:i32[])  [unwired: 4 in, 3 out]
            n113 = call-poly <vilib>:"write data element.vi"("value"=w426, "index"=w427, "data table in"=w428) -> ("data table out"=w423:T1)  [unwired: 8 in]
          }
          frame 20 {
            n114 = call-poly <vilib>:"Read.vi"("error in (no error)"=w433, "node path"=w437, "OPC UA client refnum in"=w438) -> ("error out"=w432:errorcluster, "value"=w434:u32[])  [unwired: 4 in, 3 out]
            n115 = call-poly <vilib>:"write data element.vi"("value"=w434, "index"=w435, "data table in"=w436) -> ("data table out"=w431:T1)  [unwired: 8 in]
          }
          frame 21 {
            n116 = call-poly <vilib>:"Read.vi"("error in (no error)"=w441, "node path"=w445, "OPC UA client refnum in"=w446) -> ("error out"=w440:errorcluster, "value"=w442:i64[])  [unwired: 4 in, 3 out]
            n117 = call-poly <vilib>:"write data element.vi"("value"=w442, "index"=w443, "data table in"=w444) -> ("data table out"=w439:T1)  [unwired: 8 in]
          }
          frame 22 {
            n118 = call-poly <vilib>:"Read.vi"("error in (no error)"=w449, "node path"=w453, "OPC UA client refnum in"=w454) -> ("error out"=w448:errorcluster, "value"=w450:u64[])  [unwired: 4 in, 3 out]
            n119 = call-poly <vilib>:"write data element.vi"("value"=w450, "index"=w451, "data table in"=w452) -> ("data table out"=w447:T1)  [unwired: 8 in]
          }
          frame 23 {
            n120 = call-poly <vilib>:"Read.vi"("error in (no error)"=w457, "node path"=w461, "OPC UA client refnum in"=w462) -> ("error out"=w456:errorcluster, "value"=w458:sgl[])  [unwired: 4 in, 3 out]
            n121 = call-poly <vilib>:"write data element.vi"("value"=w458, "index"=w459, "data table in"=w460) -> ("data table out"=w455:T1)  [unwired: 8 in]
          }
          frame 24 {
            n122 = call-poly <vilib>:"Read.vi"("error in (no error)"=w465, "node path"=w469, "OPC UA client refnum in"=w470) -> ("error out"=w464:errorcluster, "value"=w466:dbl[])  [unwired: 4 in, 3 out]
            n123 = call-poly <vilib>:"write data element.vi"("value"=w466, "index"=w467, "data table in"=w468) -> ("data table out"=w463:T1)  [unwired: 8 in]
          }
          frame 25 {
            n124 = call-poly <vilib>:"Read.vi"("error in (no error)"=w473, "node path"=w477, "OPC UA client refnum in"=w478) -> ("error out"=w472:errorcluster, "value"=w474:string[])  [unwired: 4 in, 3 out]
            n125 = call-poly <vilib>:"write data element.vi"("value"=w474, "index"=w475, "data table in"=w476) -> ("data table out"=w471:T1)  [unwired: 8 in]
          }
          frame 26 {
            n126 = call-poly <vilib>:"Read.vi"("error in (no error)"=w483, "node path"=w486, "OPC UA client refnum in"=w487) -> ("error out"=w482:errorcluster, "value"=w480:timestamp[])  [unwired: 4 in, 3 out]
            n127 = call "From DateTime Array.vi"("DateTime Array"=w480) -> ("Formatted DateTime Array"=w479:dbl[])
            n128 = call-poly <vilib>:"write data element.vi"("value"=w479, "index"=w484, "data table in"=w485) -> ("data table out"=w481:T1)  [unwired: 8 in]
          }
          frame 27 {
            n129 = call-poly <vilib>:"Read.vi"("error in (no error)"=w492, "node path"=w495, "OPC UA client refnum in"=w496) -> ("error out"=w491:errorcluster, "value"=w489:u8[][])  [unwired: 4 in, 3 out]
            n130 = for {
              tunnel: w489 -> [w498] mode=indexing
              tunnel: [w497] -> w488 mode=indexing
              n131 = Byte Array To String(unsigned byte array=w498) -> (string=w497:string)
            }
            n132 = call-poly <vilib>:"write data element.vi"("value"=w488, "index"=w493, "data table in"=w494) -> ("data table out"=w490:T1)  [unwired: 8 in]
          }
        }
      }
    }
  }
  "error out" <- w1
  "data table out" <- w2
  "OPC UA runtime out" <- "OPC UA runtime in"
